vi "Load Instruments.vi"(8 "Error In":errorcluster, 10 "Source":string) -> (0 "Error Out":errorcluster)   [LabVIEW 2020, in "Instrument Manager.lvclass"]
uses:
  Instrument Manager.lvclass
  Instrument Manager.lvclass/Instrument Manager.ctl
  e1c4a741-4abe-4688-a11f-f4f478980007.vi
  Config from JSON/Config from JSON.lvclass
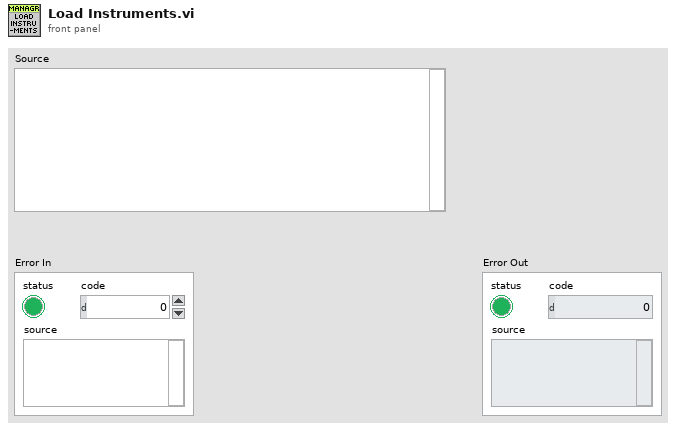
[diagram p1: front panel]
types:
  T1 = typedef "Instrument Manager.lvclass/ObjectAttributes.ctl" = cluster{"ICreate Action Point":refnum<class "ICreate Action Point.lvclass">, "IInstruments":map{string, refnum<class "IInstrument.lvclass">}, "IVirtual Instruments":map{string, refnum<class "IVirtual Instrument.lvclass">}, "Instrument Configurations":map{string, refnum<class "Config from JSON.lvclass">}, "Virtual Instrument Configurations":map{string, refnum<class "Config from JSON.lvclass">}, "Action Point Configurations":map{string, refnum<class "Config from JSON.lvclass">}, "Action Points":map{string, refnum<class "Action Point.lvclass">}}
  T2 = map{string, refnum<class "Config from JSON.lvclass">}
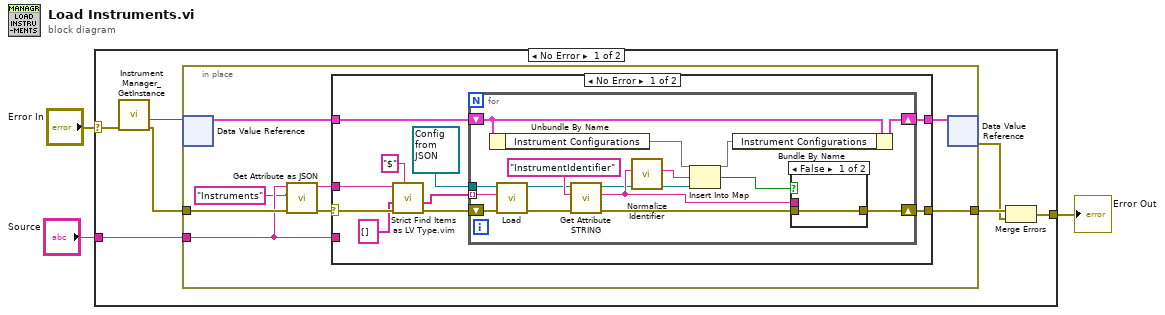
[diagram p0: block diagram]
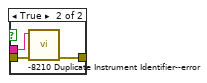
[diagram p2: hidden frame]
diagram:
  n1 = case shown="No Error" "Error In" {
    selector: "Error In" -> [w9 w51]
    tunnel: [w5 w51] -> w2
    tunnel: "Source" -> [w10 _]
    frame No Error {
      n2 = call "Instrument Manager_GetInstance.vi"("Error In"=w9) -> ("Error Out"=w8:errorcluster, "DVRRefOut"=w6:refnum<data-value>)  [unwired: 6 in, 3 out]
      n3 = in-place {
        in-place-border: w10 -> [w13]
        in-place-border: w8 -> [w18]
        in-place-border: [w15] -> w7
        n4 = in-place-dvr #1(w6) -> (w16:T1)  [unwired: 1 out]
        n5 = call "Get Attribute as JSON.vi"("error in"=w18, "Attribute"="Instruments", "Source"=w13) -> ("error out"=w17:errorcluster, "<JSON>"=w12:string)  [unwired: 7 in]
        n6 = case "Error?" shown="No Error" w17 {
          selector: w17 -> [w27 w50]
          tunnel: w16 -> [w24 w49]
          tunnel: [w23 w50] -> w15
          tunnel: [w21 w49] -> w14
          tunnel: w13 -> [_ _]
          tunnel: w12 -> [w20 _]
          frame No Error {
            n7 = call "Strict Find Items as LV Type.vim"("$Path or Item Name"="$", "error in"=w27, "Data Type and Default Value"=string[] [], "<JSON>"=w20) -> ("error out"=w25:errorcluster, "Data out"=w22:string[])  [unwired: 5 in, 1 out]
            n8 = for {
              shift-right: [w40] -> w23
              shift-left: w25 -> [w44]
              tunnel: w22 -> [w33] mode=indexing
              shift-right: [w37] -> w21
              shift-left: w24 -> [w38]
              tunnel: refnum<class "Config from JSON.lvclass"> refnum ("Config From JSON in") -> [w30]
              n9 = Unbundle By Name(w38) -> ("Instrument Configurations"=w43:T2)
              n10 = call-dynamic "Load.vi"("error in"=w44, "Source"=w33, "Config From JSON in"=w30) -> ("error out"=w34:errorcluster, "Config From JSON out"=w32:refnum<class "Config from JSON.lvclass">)  [unwired: 7 in]
              n11 = call-dynamic "Get Attribute STRING.vi"("error in"=w34, "Attribute"="InstrumentIdentifier" ("$Path or Item Name"), "ConfigFromJSON in"=w32) -> ("error out"=w41:errorcluster, "Value"=w35:string, "ConfigFromJSON out"=w31:refnum<class "Config from JSON.lvclass">)  [unwired: 6 in]
              n12 = call "Normalize Identifier.vi"("Identifier"=w35) -> ("Normalized Identifier"=w29:string)  [unwired: 10 in]
              n13 = Insert Into Map(map in=w43, key=w29, value=w31) -> (map out=w36:T2, key already included?=w39:bool)  [unwired: 1 out]
              n14 = Bundle By Name(cluster=w38, "Instrument Configurations"=w36) -> (w37:T1)
              n15 = case shown="False" w39 {
                tunnel: w41 -> [w45 w48]
                tunnel: [w45 w47] -> w40
                tunnel: w35 -> [_ w46]
                frame False {
                }
                frame True {
                  n16 = call "-8210 Duplicate Instrument Identifier--error.vi"("error in"=w48, "Instrument Identifier"=w46) -> ("error out"=w47:errorcluster)  [unwired: 9 in]
                }
              }
            }
          }
          frame Error {
          }
        }
        n17 = in-place-dvr #1(w14) -> (w4:errorcluster)  [unwired: 1 out]
      }
      n18 = Merge Errors(w7, w4) -> (w5:errorcluster)
    }
    frame Error {
    }
  }
  "Error Out" <- w2
